vi "array -- bilinear regression 2D -- V3.vi"(7 "action":T3, 9 "fit map IN":map{T2, dbl}(c390), 11 "xyzw IN":cluster{"x":dbl[], "y":dbl[], "z":dbl[]}={"x"=[-2.0, -1.0, 0.0, 1.0, 2.0], "y"=[-2.0, -1.0, 0.0, 1.0, 2.0], "z"=[12.0, 3.0, 0.0, 3.0, 12.0]}) -> (1 "fit map out":map{T2, dbl}(c390), 3 "xyzw OUT":cluster{"x":dbl[], "y":dbl[], "z":dbl[]}={"x"=[-2.0, -1.0, 0.0, 1.0, 2.0], "y"=[-2.0, -1.0, 0.0, 1.0, 2.0], "z"=[12.0, 3.0, 0.0, 3.0, 12.0]})   [LabVIEW 2021]
uses:
  array -- fit control .ctl
  array -- bilinear regression 2D.ctl
  <vilib>/Analysis/Matrix/Datatypes/RealMatrix.ctl
  <vilib>/Analysis/baseanly.llb/Matrix Type of Inverse Matrix.ctl
  <vilib>/Analysis/7linalg.llb/Solve Linear Equations (single right hand).vi
  <vilib>/Analysis/baseanly.llb/Real A x B.vi
  <vilib>/Analysis/baseanly.llb/Solve Linear Equations By Cholesky.vi
  <vilib>/Analysis/baseanly.llb/Real Matrix to Compact Array.vi
  <vilib>/Analysis/baseanly.llb/Real Compact Tri-Matrix Linear Eqs.vi
  <vilib>/Analysis/Matrix/Numeric/Conversions/Array To Matrix - RA2.vi
  <vilib>/Analysis/7linalg.llb/Solve Linear Eqs (General).vi
  <vilib>/Analysis/7linalg.llb/Solve Linear Eqs (Gen, single right hand).vi
  <vilib>/Analysis/Matrix/Numeric/Conversions/Matrix To Array - RM.vi
  <vilib>/Analysis/NI_AALBase.lvlib
  <vilib>/Analysis/Matrix/NI_Matrix.lvlib
  <vilib>/Analysis/NI_AALPro.lvlib
panel:
  out "subarray":dbl[](array[numeric])
  out "Real Matrix":T1
  out "fit  IN":dbl[](array[numeric])=[1.9, 2.6, 3.3, 1.0, 2.7, 3.9]
  out "fit OUT":dbl[](array[numeric])=[1.0, 1.0, 1.0, 0.0, 0.0, 0.0]
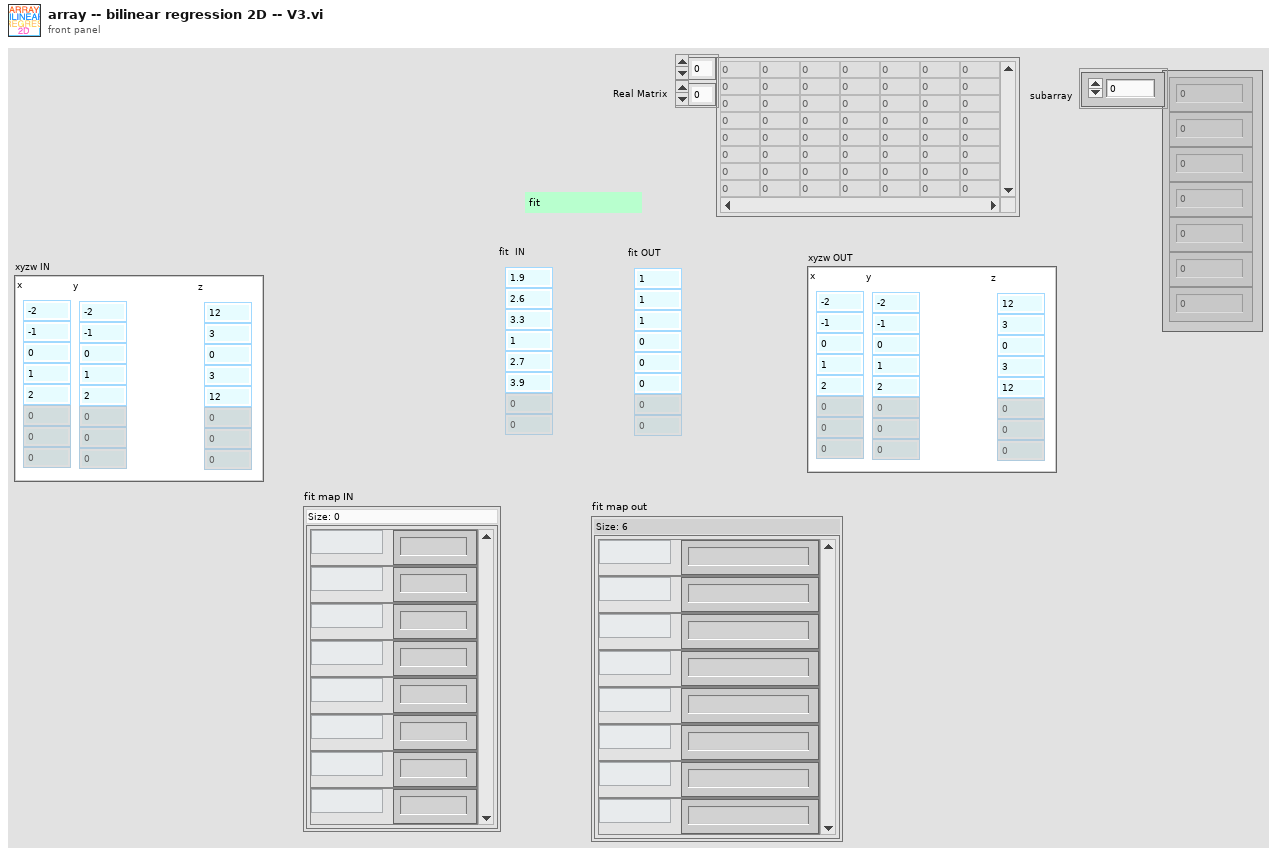
[diagram p1: front panel]
types:
  T1 = typedef "NI_Matrix.lvlib/RealMatrix.ctl" = dbl[][]
  T2 = typedef "array -- bilinear regression 2D.ctl" = enum16{"1", "x", "y", "xx", "xy", "yy", "xxy", "xyy", "yyy", "xxx", "xxyy", "xyyy", "xxxy", "yyyy", "xxxx", "xxz", "xyz", "yyz", "xz", "yz", "z", "wwz", "ywz", "xwz", "xxxw", "xxyw", "xyyw", "yyyw", "xxww", "xyww", "yyww", "xwww", "ywww", "wwww", "ww", "xw", "yw", "w", "wz"}
  T3 = typedef "array -- fit control .ctl" = enum16{"fit", "calc", "check", "init"}
  T4 = typedef "NI_AALBase.lvlib/Matrix Type of Inverse Matrix.ctl" = enum32{"General", "Positive Definite", "Lower Triangular", "Upper Triangular"}
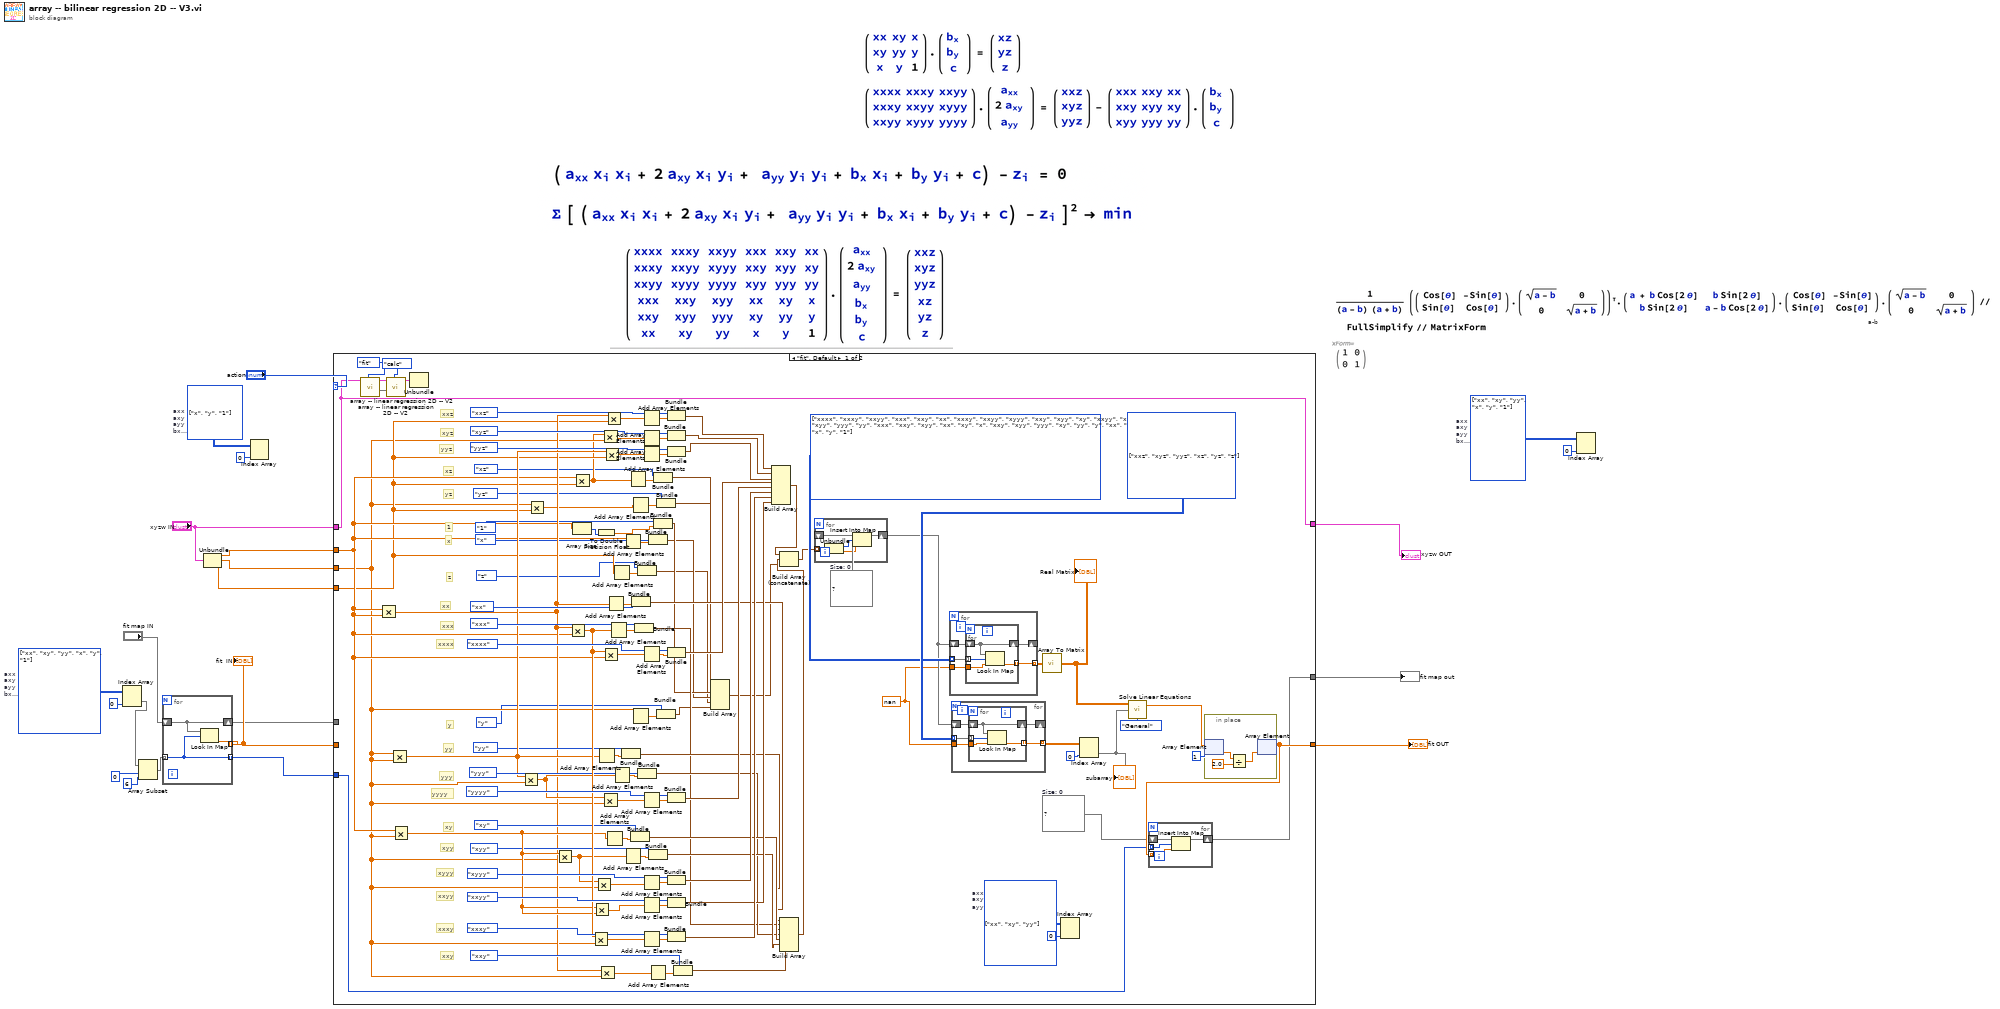
[diagram p0: block diagram]
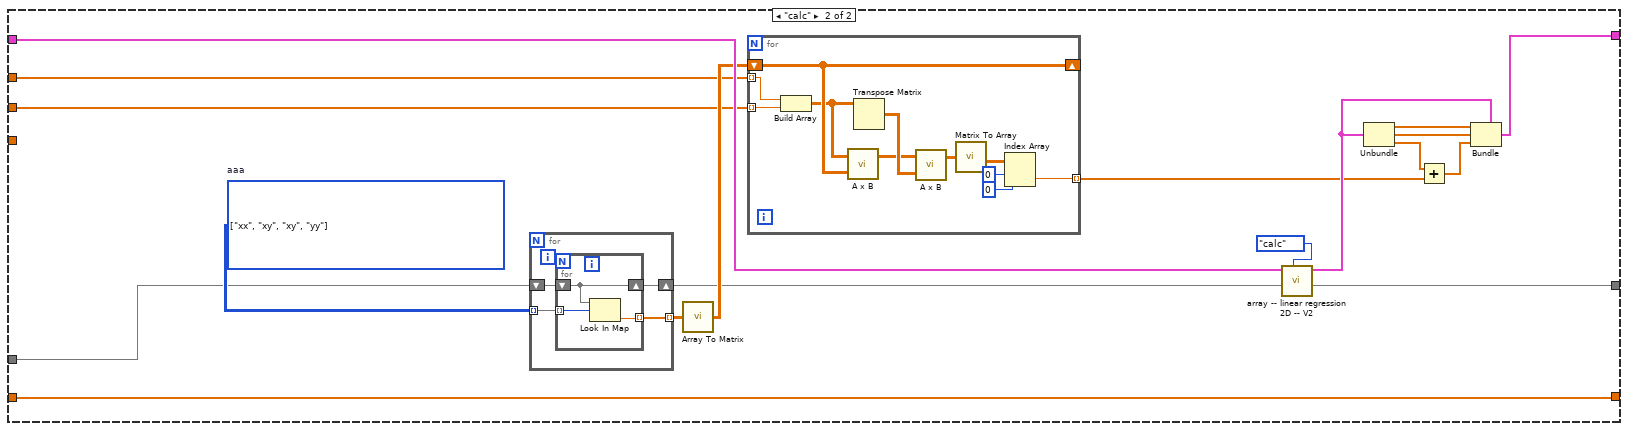
[diagram p2: hidden frame]
diagram:
  w12 = T2[][] [[enum."x"], [enum."y"], [enum."1"]] items=["1", "x", "y", "xx", "xy", "yy", "xxy", "xyy", "yyy", "xxx", "xxyy", "xyyy", "xxxy", "yyyy", "xxxx", "xxz", "xyz", "yyz", "xz", "yz", "z", "wwz", "ywz", "xwz", "xxxw", "xxyw", "xyyw", "yyyw", "xxww", "xyww", "yyww", "xwww", "ywww", "wwww", "ww", "xw", "yw", "w", "wz"]  # axx axy ayy bx by c
  w16 = T2[][] [[enum."xx"], [enum."xy"], [enum."yy"], [enum."x"], [enum."y"], [enum."1"]] items=["1", "x", "y", "xx", "xy", "yy", "xxy", "xyy", "yyy", "xxx", "xxyy", "xyyy", "xxxy", "yyyy", "xxxx", "xxz", "xyz", "yyz", "xz", "yz", "z", "wwz", "ywz", "xwz", "xxxw", "xxyw", "xyyw", "yyyw", "xxww", "xyww", "yyww", "xwww", "ywww", "wwww", "ww", "xw", "yw", "w", "wz"]  # axx axy ayy bx by c
  w18 = T2[][] [[enum."xx"], [enum."xy"], [enum."yy"], [enum."x"], [enum."y"], [enum."1"]] items=["1", "x", "y", "xx", "xy", "yy", "xxy", "xyy", "yyy", "xxx", "xxyy", "xyyy", "xxxy", "yyyy", "xxxx", "xxz", "xyz", "yyz", "xz", "yz", "z", "wwz", "ywz", "xwz", "xxxw", "xxyw", "xyyw", "yyyw", "xxww", "xyww", "yyww", "xwww", "ywww", "wwww", "ww", "xw", "yw", "w", "wz"]  # axx axy ayy bx by c
  # "a-b"
  n1 = Index Array(array=w16, index (col)=0 ("disabled index (col)")) -> (element=w7:T2[])  [unwired: 1 in]
  n2 = Array Subset(array=w7, index=0 ("disabled index (col)"), length=6) -> (w4:T2[])
  n3 = for {
    shift-right: [w24] -> w10
    shift-left: "fit map IN" -> [w24]
    tunnel: w4 -> [w23] mode=indexing
    tunnel: [w25] -> w13 mode=indexing
    tunnel: [w23] -> w3 mode=indexing
    n4 = Look In Map(map=w24, key=w23) -> (value=w25:dbl)  [unwired: 1 in, 1 out]
  }
  "fit  IN" <- w13
  n5 = Unbundle("xyzw IN") -> ("x"=w21:dbl[], "y"=w20:dbl[], "z"=w9:dbl[])
  n6 = Index Array(array=w12, index (col)=0 ("disabled index (col)")) -> ()  [unwired: 1 in, 1 out]
  n7 = case shown="\"fit\", Default" "action" {
    tunnel: w9 -> [w44 _]
    tunnel: w21 -> [w47 w169]
    tunnel: [w106 w186] -> w19
    tunnel: w13 -> [_ w186]
    tunnel: w20 -> [w41 w177]
    tunnel: w10 -> [_ w179]
    tunnel: "xyzw IN" -> [w92 w184]
    tunnel: [w93 w183] -> w8
    tunnel: [w92 w170] -> w1
    tunnel: w3 -> [w91 _]
    frame "fit", Default {
      w26 = map{T2, dbl} {}  # Size: 0
      w27 = nan ("default value")
      w95 = T2[][] [[enum."xx"], [enum."xy"], [enum."yy"]] items=["1", "x", "y", "xx", "xy", "yy", "xxy", "xyy", "yyy", "xxx", "xxyy", "xyyy", "xxxy", "yyyy", "xxxx", "xxz", "xyz", "yyz", "xz", "yz", "z", "wwz", "ywz", "xwz", "xxxw", "xxyw", "xyyw", "yyyw", "xxww", "xyww", "yyww", "xwww", "ywww", "wwww", "ww", "xw", "yw", "w", "wz"]  # axx axy ayy
      w105 = T2[][] [[enum."xxz"], [enum."xyz"], [enum."yyz"], [enum."xz"], [enum."yz"], [enum."z"]] items=["1", "x", "y", "xx", "xy", "yy", "xxy", "xyy", "yyy", "xxx", "xxyy", "xyyy", "xxxy", "yyyy", "xxxx", "xxz", "xyz", "yyz", "xz", "yz", "z", "wwz", "ywz", "xwz", "xxxw", "xxyw", "xyyw", "yyyw", "xxww", "xyww", "yyww", "xwww", "ywww", "wwww", "ww", "xw", "yw", "w", "wz"]
      w104 = T2[][] [[enum."xxxx", enum."xxxy", enum."xxyy", enum."xxx", enum."xxy", enum."xx"], [enum."xxxy", enum."xxyy", enum."xyyy", enum."xxy", enum."xyy", enum."xy"], [enum."xxyy", enum."xyyy", enum."yyyy", enum."xyy", enum."yyy", enum."yy"], [enum."xxx", enum."xxy", enum."xyy", enum."xx", enum."xy", enum."x"], [enum."xxy", enum."xyy", enum."yyy", enum."xy", enum."yy", enum."y"], [enum."xx", enum."xy", enum."yy", enum."x", enum."y", enum."1"]] items=["1", "x", "y", "xx", "xy", "yy", "xxy", "xyy", "yyy", "xxx", "xxyy", "xyyy", "xxxy", "yyyy", "xxxx", "xxz", "xyz", "yyz", "xz", "yz", "z", "wwz", "ywz", "xwz", "xxxw", "xxyw", "xyyw", "yyyw", "xxww", "xyww", "yyww", "xwww", "ywww", "wwww", "ww", "xw", "yw", "w", "wz"]
      w107 = map{T2, dbl} {}  # Size: 0
      # "z"
      # "xxz"
      # "yz"
      # "xz"
      # "yyz"
      # "xyz"
      # "xxy"
      # "xxxy"
      # "xxyy"
      # "xyyy"
      # "xyy"
      # "xy"
      # "yyyy"
      # "yyy"
      # "yy"
      # "y"
      # "1"
      # "xxxx"
      # "xxx"
      # "xx"
      # "x"
      n8 = call "array -- linear regression 2D -- V2.vi"("action"=array_--_fit_control_."fit", "xyz IN"=w92) -> ("fit map out"=w99:map{T2, dbl}, "xyz OUT"=w98:cluster{"x":dbl[], "y":dbl[], "z":dbl[]})  [unwired: 8 in]
      n9 = Multiply(x=w47, y=w47) -> (x*y=w63:dbl[])
      n10 = call "array -- linear regression 2D -- V2.vi"("action"=array_--_fit_control_."calc", "fit map IN"=w99, "xyz IN"=w98) -> ("xyz OUT"=w100:cluster{"x":dbl[], "y":dbl[], "z":dbl[]})  [unwired: 7 in, 1 out]
      n11 = Multiply(x=w41, y=w41) -> (x*y=w68:dbl[])
      n12 = Multiply(x=w47, y=w41) -> (x*y=w76:dbl[])
      n13 = Unbundle(w100) -> ()  [unwired: 3 out]
      n14 = Multiply(x=w68, y=w41) -> (x*y=w79:dbl[])
      n15 = Multiply(x=w41, y=w44) -> (x*y=w52:dbl[])
      n16 = Multiply(x=w76, y=w41) -> (x*y=w73:dbl[])
      n17 = Multiply(x=w63, y=w47) -> (x*y=w82:dbl[])
      n18 = Array Size(array=w47) -> (size(s)=w34:i32)
      n19 = Multiply(x=w47, y=w44) -> (x*y=w38:dbl[])
      n20 = Multiply(x=w82, y=w41) -> (x*y=w134:dbl[])
      n21 = Multiply(x=w76, y=w76) -> (x*y=w135:dbl[])
      n22 = Multiply(x=w73, y=w41) -> (x*y=w136:dbl[])
      n23 = To Double Precision Float(number=w34) -> (double precision float=w33:dbl)
      n24 = Add Array Elements(numeric array=w68) -> (sum=w69:dbl)
      n25 = Multiply(x=w63, y=w41) -> (x*y=w66:dbl[])
      n26 = Multiply(x=w38, y=w41) -> (x*y=w131:dbl[])
      n27 = Multiply(x=w79, y=w41) -> (x*y=w137:dbl[])
      n28 = Multiply(x=w82, y=w47) -> (x*y=w138:dbl[])
      n29 = Multiply(x=w68, y=w44) -> (x*y=w133:dbl[])
      n30 = Multiply(x=w63, y=w44) -> (x*y=w132:dbl[])
      n31 = Add Array Elements(numeric array=w76) -> (sum=w77:dbl)
      n32 = Add Array Elements(numeric array=w63) -> (sum=w71:dbl)
      n33 = Add Array Elements(numeric array=w82) -> (sum=w83:dbl)
      n34 = Add Array Elements(numeric array=w44) -> (sum=w45:dbl)
      n35 = Add Array Elements(numeric array=w79) -> (sum=w80:dbl)
      n36 = Bundle(array_--_bilinear_regression_2D."yy", "Numeric"=w69) -> (w58:cluster{T2, "Numeric":dbl})  [unwired: 1 in]
      n37 = Add Array Elements(numeric array=w47) -> (sum=w48:dbl)
      n38 = Add Array Elements(numeric array=w73) -> (sum=w74:dbl)
      n39 = Add Array Elements(numeric array=w38) -> (sum=w39:dbl)
      n40 = Bundle(array_--_bilinear_regression_2D."xy", "Numeric"=w77) -> (w60:cluster{T2, "Numeric":dbl})  [unwired: 1 in]
      n41 = Add Array Elements(numeric array=w52) -> (sum=w51:dbl)
      n42 = Add Array Elements(numeric array=w41) -> (sum=w42:dbl)
      n43 = Bundle(array_--_bilinear_regression_2D."xx", "Numeric"=w71) -> (w56:cluster{T2, "Numeric":dbl})  [unwired: 1 in]
      n44 = Bundle(array_--_bilinear_regression_2D."xxx", "Numeric"=w83) -> (w57:cluster{T2, "Numeric":dbl})  [unwired: 1 in]
      n45 = Bundle(array_--_bilinear_regression_2D."z", "Numeric"=w45) -> (w30:cluster{T2, "Numeric":dbl})  [unwired: 1 in]
      n46 = Bundle(array_--_bilinear_regression_2D."yyy", "Numeric"=w80) -> (w59:cluster{T2, "Numeric":dbl})  [unwired: 1 in]
      n47 = Add Array Elements(numeric array=w132) -> (sum=w130:dbl)
      n48 = Add Array Elements(numeric array=w131) -> (sum=w128:dbl)
      n49 = Add Array Elements(numeric array=w133) -> (sum=w125:dbl)
      n50 = Add Array Elements(numeric array=w138) -> (sum=w115:dbl)
      n51 = Add Array Elements(numeric array=w137) -> (sum=w118:dbl)
      n52 = Add Array Elements(numeric array=w136) -> (sum=w120:dbl)
      n53 = Add Array Elements(numeric array=w135) -> (sum=w122:dbl)
      n54 = Add Array Elements(numeric array=w134) -> (sum=w124:dbl)
      n55 = Bundle(array_--_bilinear_regression_2D."x", "Numeric"=w48) -> (w31:cluster{T2, "Numeric":dbl})  [unwired: 1 in]
      n56 = Bundle(array_--_bilinear_regression_2D."xyy", "Numeric"=w74) -> (w61:cluster{T2, "Numeric":dbl})  [unwired: 1 in]
      n57 = Add Array Elements(numeric array=w66) -> (sum=w65:dbl)
      n58 = Bundle(array_--_bilinear_regression_2D."xz", "Numeric"=w39) -> (w36:cluster{T2, "Numeric":dbl})  [unwired: 1 in]
      n59 = Bundle(array_--_bilinear_regression_2D."1", w33) -> (w32:cluster{T2, dbl})  [unwired: 1 in]
      n60 = Bundle(array_--_bilinear_regression_2D."yz", "Numeric"=w51) -> (w35:cluster{T2, "Numeric":dbl})  [unwired: 1 in]
      n61 = Bundle(array_--_bilinear_regression_2D."y", "Numeric"=w42) -> (w29:cluster{T2, "Numeric":dbl})  [unwired: 1 in]
      n62 = Bundle(array_--_bilinear_regression_2D."xxz", "Numeric"=w130) -> (w101:cluster{T2, "Numeric":dbl})  [unwired: 1 in]
      n63 = Bundle(array_--_bilinear_regression_2D."xyz", "Numeric"=w128) -> (w102:cluster{T2, "Numeric":dbl})  [unwired: 1 in]
      n64 = Bundle(array_--_bilinear_regression_2D."yyz", "Numeric"=w125) -> (w103:cluster{T2, "Numeric":dbl})  [unwired: 1 in]
      n65 = Bundle(array_--_bilinear_regression_2D."xxxx", "Numeric"=w115) -> (w114:cluster{T2, "Numeric":dbl})  [unwired: 1 in]
      n66 = Bundle(array_--_bilinear_regression_2D."yyyy", "Numeric"=w118) -> (w113:cluster{T2, "Numeric":dbl})  [unwired: 1 in]
      n67 = Bundle(array_--_bilinear_regression_2D."xyyy", "Numeric"=w120) -> (w112:cluster{T2, "Numeric":dbl})  [unwired: 1 in]
      n68 = Bundle(array_--_bilinear_regression_2D."xxyy", "Numeric"=w122) -> (w110:cluster{T2, "Numeric":dbl})  [unwired: 1 in]
      n69 = Bundle(array_--_bilinear_regression_2D."xxxy", "Numeric"=w124) -> (w111:cluster{T2, "Numeric":dbl})  [unwired: 1 in]
      n70 = Bundle(array_--_bilinear_regression_2D."xxy", "Numeric"=w65) -> (w62:cluster{T2, "Numeric":dbl})  [unwired: 1 in]
      n71 = Build Array(w36, w35, w32, w31, w30, w29) -> (w28:cluster{T2, "Numeric":dbl}[])
      n72 = Build Array(w101, w102, w103, w114, w113, w112, w111, w110) -> (w55:cluster{T2, "Numeric":dbl}[])
      n73 = Build Array(w56, w57, w58, w59, w60, w61, w62) -> (w54:cluster{T2, "Numeric":dbl}[])
      n74 = Build Array (concatenate)(w55, w54, w28) -> (w53:cluster{T2, "Numeric":dbl}[])
      n75 = for {
        tunnel: w53 -> [w157] mode=indexing
        shift-right: [w158] -> w85
        shift-left: w107 -> [w159]
        n76 = Unbundle(w157) -> (w156:T2, "Numeric"=w155:dbl)
        n77 = Insert Into Map(map in=w159, key=w156, value=w155) -> (map out=w158:map{T2, dbl})  [unwired: 2 out]
      }
      n78 = for {
        tunnel: w104 -> [w164] mode=indexing
        shift-right: [w162] -> _
        shift-left: w85 -> [w163]
        tunnel: [w161] -> w109 mode=indexing
        tunnel: w27 -> [w160]
        n79 = for {
          tunnel: w164 -> [w167] mode=indexing
          shift-right: [w168] -> w162
          shift-left: w163 -> [w168]
          tunnel: [w166] -> w161 mode=indexing
          tunnel: w160 -> [w165]
          n80 = Look In Map(map=w168, key=w167, default value=w165) -> (value=w166:dbl)  [unwired: 1 out]
        }
      }
      n81 = for {
        shift-right: [w149] -> _
        shift-left: w85 -> [w150]
        tunnel: w105 -> [w148] mode=indexing
        tunnel: [w147] -> w84 mode=indexing
        tunnel: w27 -> [w146]
        n82 = for {
          shift-right: [w154] -> w149
          shift-left: w150 -> [w154]
          tunnel: w148 -> [w153] mode=indexing
          tunnel: [w152] -> w147 mode=indexing
          tunnel: w146 -> [w151]
          n83 = Look In Map(map=w154, key=w153, default value=w151) -> (value=w152:dbl)  [unwired: 1 out]
        }
      }
      n84 = call-poly <vilib>:"Array To Matrix.vi"("Real 2D Array"=w109) -> ("Real Matrix"=w87:T1)
      "Real Matrix" <- w87
      n85 = Index Array(array=w95, index (col)=0 ("disabled index (col)")) -> ()  [unwired: 1 in, 1 out]
      n86 = Index Array(array=w84, index (col)=0 ("disabled index (col)")) -> (element=w89:dbl[])  [unwired: 1 in]
      "subarray" <- w89
      n87 = call-poly <vilib>:"Solve Linear Equations.vi"("matrix type"=Matrix_Type_of_Inverse_Matrix."General", "Known Vector"=w89, "Input Matrix"=w87) -> ("Solution Vector"=w86:dbl[])  [unwired: 1 out]
      n88 = in-place {
        n89 = in-place-array #1(w86, 1) -> (w145:dbl)
        n90 = Divide(x=w145, y=2.0) -> (x/y=w143:dbl)
        n91 = in-place-array #1(w143) -> (w106:dbl[])  [unwired: 1 out]
      }
      n92 = for {
        shift-right: [w141] -> w93
        shift-left: w26 -> [w142]
        tunnel: w91 -> [w140] mode=indexing
        tunnel: w106 -> [w139] mode=indexing
        n93 = Insert Into Map(map in=w142, key=w140, value=w139) -> (map out=w141:map{T2, dbl})  [unwired: 2 out]
      }
    }
    frame "calc" {
      w181 = T2[][] [[enum."xx", enum."xy"], [enum."xy", enum."yy"]] items=["1", "x", "y", "xx", "xy", "yy", "xxy", "xyy", "yyy", "xxx", "xxyy", "xyyy", "xxxy", "yyyy", "xxxx", "xxz", "xyz", "yyz", "xz", "yz", "z", "wwz", "ywz", "xwz", "xxxw", "xxyw", "xyyw", "yyyw", "xxww", "xyww", "yyww", "xwww", "ywww", "wwww", "ww", "xw", "yw", "w", "wz"]  # aaa
      n94 = for {
        tunnel: w181 -> [w201] mode=indexing
        shift-right: [w199] -> w178
        shift-left: w179 -> [w200]
        tunnel: [w198] -> w182 mode=indexing
        n95 = for {
          tunnel: w201 -> [w203] mode=indexing
          shift-right: [w204] -> w199
          shift-left: w200 -> [w204]
          tunnel: [w202] -> w198 mode=indexing
          n96 = Look In Map(map=w204, key=w203) -> (value=w202:dbl)  [unwired: 1 in, 1 out]
        }
      }
      n97 = call-poly <vilib>:"Array To Matrix.vi"("Real 2D Array"=w182) -> ("Real Matrix"=w180:T1)
      n98 = for {
        tunnel: w177 -> [w196] mode=indexing
        shift-right: [w195] -> _
        shift-left: w180 -> [w195]
        tunnel: [w188] -> w171 mode=indexing
        tunnel: w169 -> [w187] mode=indexing
        n99 = Build Array(w187, w196) -> (w194:T1)
        n100 = call-poly <vilib>:"A x B.vi"("B"=w195, "A"=w194) -> ("A x B"=w192:T1)  [unwired: 1 out]
        n101 = Transpose Matrix(1:w194) -> (0:w193:T1)
        n102 = call-poly <vilib>:"A x B.vi"("B"=w193, "A"=w192) -> ("A x B"=w197:T1)  [unwired: 1 out]
        n103 = call-poly <vilib>:"Matrix To Array.vi"("Real Matrix"=w197) -> ("Real 2D Array"=w191:dbl[][])
        n104 = Index Array(array=w191, index (row)=0, index (col)=0 ("disabled index (col)")) -> (element=w188:dbl)
      }
      n105 = call "array -- linear regression 2D -- V2.vi"("action"=array_--_fit_control_."calc", "fit map IN"=w178, "xyz IN"=w184) -> ("fit map out"=w183:map{T2, dbl}, "xyz OUT"=w172:cluster{"x":dbl[], "y":dbl[], "z":dbl[]})  [unwired: 7 in]
      n106 = Unbundle(w172) -> ("x"=w176:dbl[], "y"=w175:dbl[], "z"=w174:dbl[])
      n107 = Add(x=w174, y=w171) -> (x+y=w173:dbl[])
      n108 = Bundle(cluster=w172, "x"=w176, "y"=w175, "z"=w173) -> (w170:cluster{"x":dbl[], "y":dbl[], "z":dbl[]})
    }
  }
  "fit OUT" <- w19
  "fit map out" <- w8
  "xyzw OUT" <- w1
  n109 = Index Array(array=w18, index (col)=0 ("disabled index (col)")) -> ()  [unwired: 1 in, 1 out]
